vi "timestampTest.vi"   [LabVIEW 2016]
uses:
  Common_FPGA_Timestamp/FPGATimestamp.lvlib
  Common_FPGA_Timestamp/DataTypes/TimestampSettings.ctl
  <vilib>/rvi/DataTransferAndStorage/Container/XNode/niFpgaContainer.xnode
  <vilib>/rvi/DataTransferAndStorage/Register/Emulation/niFpgaRegisterEmulation.vi
  <vilib>/rvi/interface/RandomDataEmulation/nirviRandomDataFpgaReadWriteTemplate.vi
types:
  T1 = typedef "FPGATimestamp.lvlib/TimestampSettings.ctl" = cluster{"TimeRegister":refnum<k21>, "TimeSource":refnum<k21>, "IterationsPerMicrosecond":i16, "UpdateFIFO":refnum<k21>}
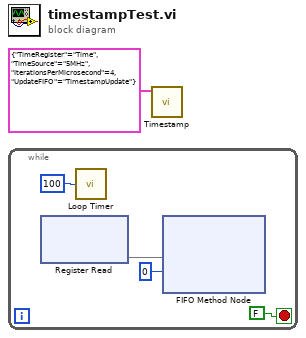
[diagram p0: block diagram]
diagram:
  n1 = while {
    stop <- FALSE stop-if-true
    n2 = xnode ("Register Read")() -> ("Data"=w2)  [unwired: 1 in, 1 out]
    n3 = call "Loop Timer"("Count(mSec)"=u32 100) -> ()  [unwired: 1 out]
    n4 = xnode ("FIFO Method Node")("Element"=w2, "Timeout"=0) -> ()  [unwired: 1 in, 2 out]
  }
  n5 = call "Timestamp.vi"("TimestampSettings"=T1 {"TimeRegister"="Time", "TimeSource"="5MHz", "IterationsPerMicrosecond"=4, "UpdateFIFO"="TimestampUpdate"}) -> ()  [unwired: 11 in]
